vi "UR_task_generator.vi"() -> (1 "Tool Out":string, 2 "String":string, 3 "Task Out":string)   [LabVIEW 2022 SP3]
panel:
  in  "Insect-data-array (out of range removed)  2":dbl[][](array[numeric])
  in  "Numeric":i32
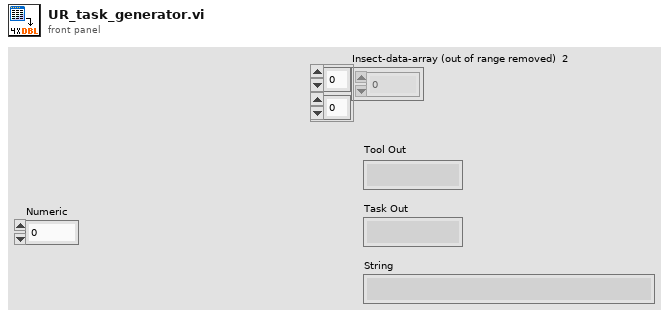
[diagram p1: front panel]
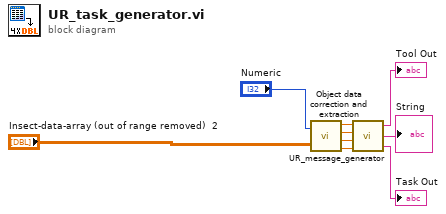
[diagram p0: block diagram]
diagram:
  n1 = call "Object data correction and extraction.vi"("Object number of interest"="Numeric", "Object-data-array"="Insect-data-array (out of range removed)  2") -> ("Obejct length"=w8:dbl, "Object CoM X"=w6:dbl, "Obejct CoM Y"=w5:dbl, "Object orientation"=w9:dbl)
  n2 = call "UR_message_generator.vi"("Object orientation"=w9, "Obejct CoM Y"=w5, "Object CoM X"=w6, "Obejct length"=w8) -> ("Task Out"=→"Task Out":string, "UR message"=→"String":string, "Tool Out"=→"Tool Out":string)
